vi "Write Card Reader.vi"(8 "error in (no error)":errorcluster, 10 "Card Reader":bool, 11 "Simulated User Console Actor in":refnum<class "Simulated User Console Actor.lvclass">) -> (0 "error out":errorcluster, 3 "Simulated User Console Actor out":refnum<class "Simulated User Console Actor.lvclass">)   [LabVIEW 2019, in "Simulated User Console Actor.lvlib" / "Simulated User Console Actor.lvclass"]
uses:
  Simulated User Console Actor.lvclass
  Simulated User Console Actor.lvclass/Simulated User Console Actor.ctl
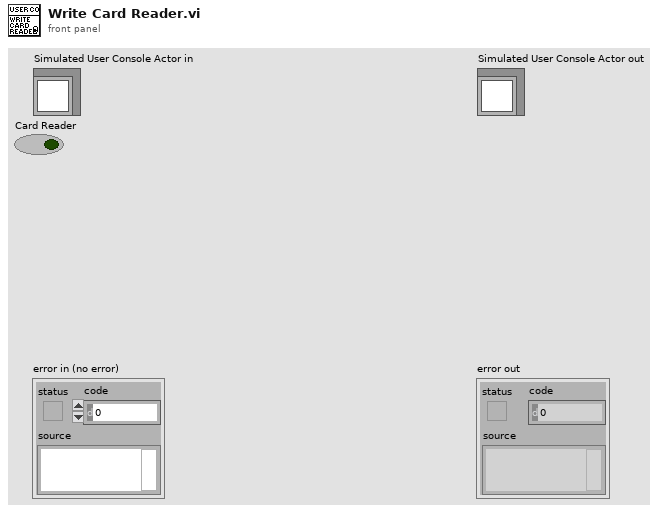
[diagram p1: front panel]
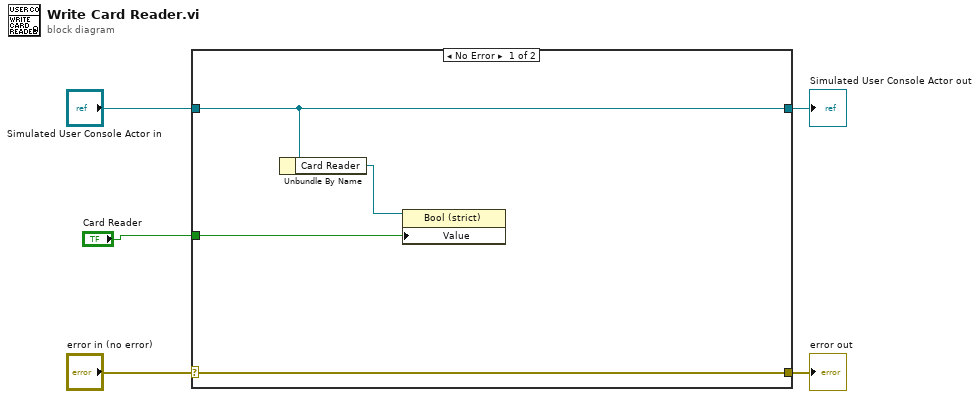
[diagram p0: block diagram]
diagram:
  n1 = case shown="No Error" "error in (no error)" {
    selector: "error in (no error)" -> [w9 w11]
    tunnel: [w9 w11] -> w4
    tunnel: [w8 w10] -> w2
    tunnel: "Simulated User Console Actor in" -> [w8 w10]
    tunnel: "Card Reader" -> [w6 _]
    frame No Error {
      n2 = Unbundle By Name(w8) -> ("Card Reader"=w7:refnum<vi>)
      n3 = property class="Bool (strict)"(reference=w7, "Value"=w6) -> ()  [unwired: 1 in, 2 out]
    }
    frame Error {
    }
  }
  "error out" <- w4
  "Simulated User Console Actor out" <- w2
